vi "ViperHawk Save Search Parameter File.vi"(10 "Debug Search Parameters":T1={"Pause"=["MchStdby", "MchPz", "MchIdl", "Machine Standby", "Machine Pause", "Machine Idle"], "Run"=["MchRn", "Machine Run", "Resume Process"], "EOC"=["EOC"], "Error Codes"=["Error1", "try", "rty", "inverr"]}, 11 "Configuration Path":path) -> ()   [LabVIEW 2016]
uses:
  Type Definitions/ViperHawk/ViperHawk Search Control.ctl
  <vilib>/Utility/file.llb/Read From Spreadsheet File (string).vi
  <vilib>/Utility/file.llb/Write To Spreadsheet File (string).vi
panel:
  out "output array":string[][](array[string])
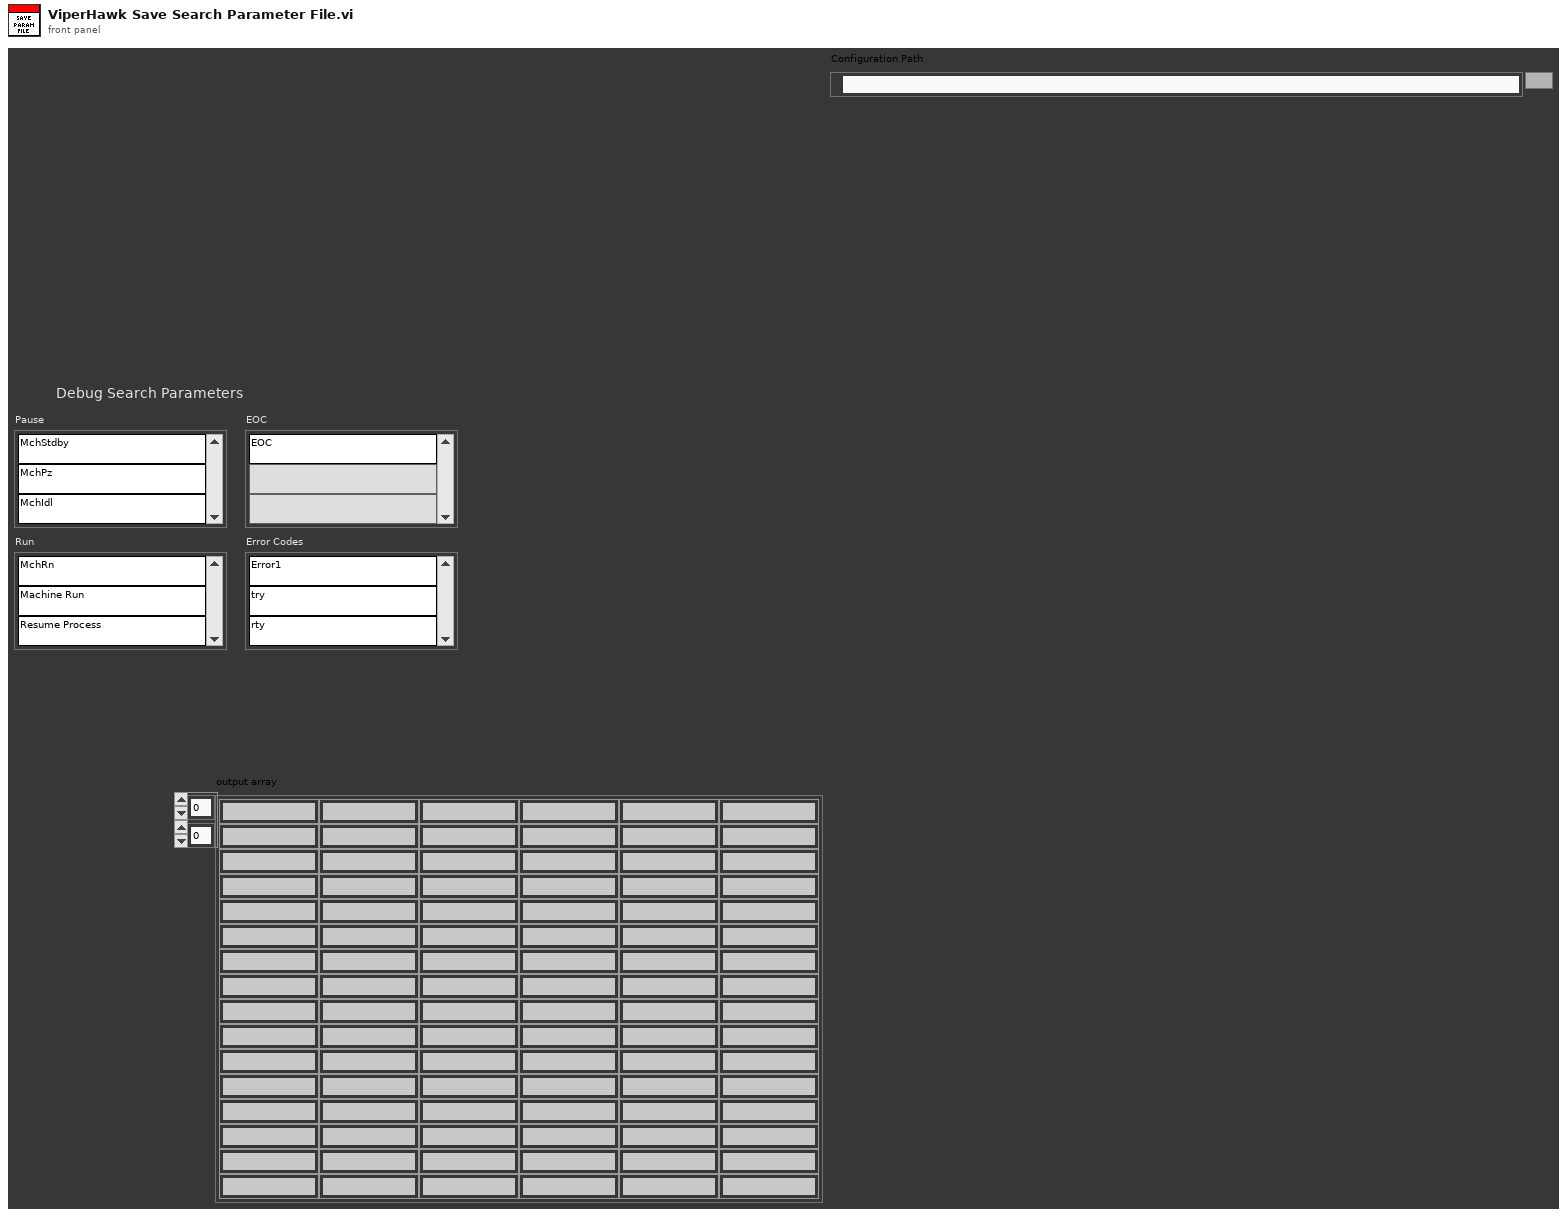
[diagram p1: front panel]
types:
  T1 = typedef "ViperHawk Search Control.ctl" = cluster{"Pause":string[], "Run":string[], "EOC":string[], "Error Codes":string[]}
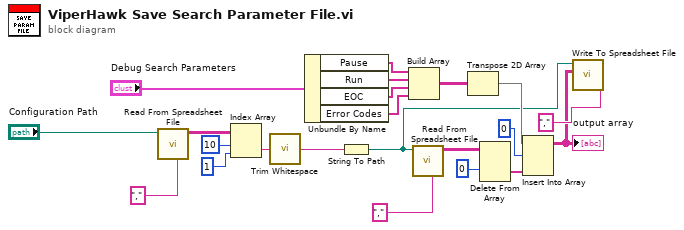
[diagram p0: block diagram]
diagram:
  n1 = call-poly <vilib>:"Read From Spreadsheet File.vi"("delimiter (\\t)"="," ("delimiter (\\t)"), "file path (dialog if empty)"="Configuration Path") -> ("all rows"=w20:string[][])  [unwired: 5 in, 4 out]
  n2 = Index Array(array=w20, index (row)=10, index (col)=1) -> (element=w17:string)
  n3 = call <vilib>:"Trim Whitespace.vi"("string"=w17) -> ("trimmed string"=w16:string)  [unwired: 1 in]
  n4 = Unbundle By Name("Debug Search Parameters") -> ("Pause"=w11:string[], "Run"=w10:string[], "EOC"=w9:string[], "Error Codes"=w8:string[])
  n5 = String To Path(string=w16) -> (path=w3:path)
  n6 = Build Array(w11, w10, w9, w8) -> (w7:string[][])
  n7 = call-poly <vilib>:"Read From Spreadsheet File.vi"("delimiter (\\t)"="," ("delimiter (\\t)"), "file path (dialog if empty)"=w3) -> ("all rows"=w14:string[][])  [unwired: 5 in, 4 out]
  n8 = Transpose 2D Array(2D array=w7) -> (transposed array=w6:string[][])
  n9 = Delete From Array(array=w14, index (row)=0) -> (deleted portion=w5:string[])  [unwired: 2 in, 1 out]
  n10 = Insert Into Array(array=w6, index (row)=0, new element=w5) -> (w1:string[][])  [unwired: 1 in]
  "output array" <- w1
  n11 = call-poly <vilib>:"Write To Spreadsheet File.vi"("delimiter (\\t)"="," ("delimiter (\\t)"), "2D data"=w1, "file path (dialog if empty)"=w3) -> ()  [unwired: 5 in, 1 out]
